vi "Set_init_data.vi"(8 "error in (no error)":errorcluster, 11 "HIS in":refnum<class "HIS.lvclass">) -> (0 "error out":errorcluster, 3 "HIS out":refnum<class "HIS.lvclass">)   [LabVIEW 2018, in "HIS.lvclass"]
uses:
  HIS.lvclass
  C:/Users/Sergey Denisov/Documents/REPS/TRANCON/Classes/DATA/DATA.lvclass
  DATA.lvclass/DATA.ctl
  Write width, pixels.vi
  Write height, pixels.vi
  DATA.lvclass
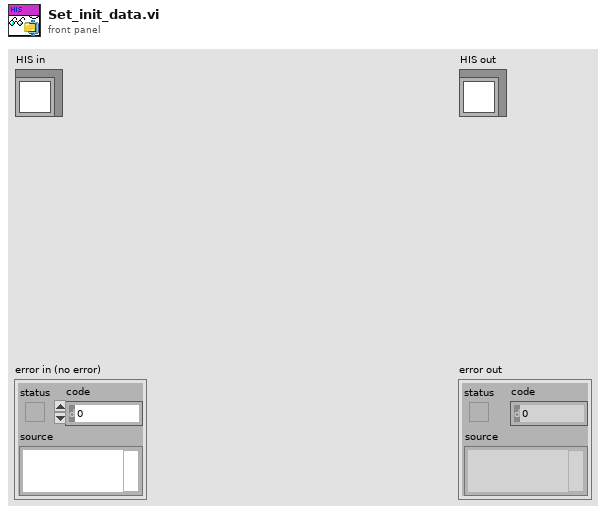
[diagram p1: front panel]
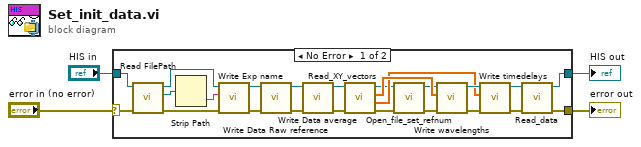
[diagram p0: block diagram]
diagram:
  n1 = case shown="No Error" "error in (no error)" {
    selector: "error in (no error)" -> [w28 w30]
    tunnel: [w5 w30] -> w3
    tunnel: "HIS in" -> [w27 w29]
    tunnel: [w6 w29] -> w1
    frame No Error {
      n2 = call "Read FilePath.vi"("error in (no error)"=w28, "DATA in"=w27) -> ("error out"=w25:errorcluster, "FilePath"=w24:path, "DATA out"=w22:refnum<class "HIS.lvclass">)  [unwired: 7 in]
      n3 = Strip Path(path=w24) -> (name=w23:string)  [unwired: 1 out]
      n4 = call "Write Exp name.vi"("error in (no error)"=w25, "Exp name"=w23, "DATA in"=w22) -> ("error out"=w20:errorcluster, "DATA out"=w19:refnum<class "HIS.lvclass">)  [unwired: 7 in]
      n5 = call "Write Data Raw reference.vi"("error in (no error)"=w20, "DATA in"=w19) -> ("error out"=w18:errorcluster, "DATA out"=w17:refnum<class "HIS.lvclass">)  [unwired: 8 in]
      n6 = call "Write Data average.vi"("error in (no error)"=w18, "DATA in"=w17) -> ("error out"=w16:errorcluster, "DATA out"=w15:refnum<class "HIS.lvclass">)  [unwired: 8 in]
      n7 = call-dynamic "Read_XY_vectors.vi"("error in (no error)"=w16, "HIS in"=w15) -> ("error out"=w12:errorcluster, "timedelays"=w13:dbl[], "wavelengths"=w14:dbl[], "HIS out"=w11:refnum<class "HIS.lvclass">)  [unwired: 6 in]
      n8 = call-dynamic "Open_file_set_refnum.vi"("error in (no error)"=w12, "DATA in"=w11) -> ("error out"=w10:errorcluster, "DATA out"=w9:refnum<class "HIS.lvclass">)  [unwired: 8 in]
      n9 = call "Write wavelengths.vi"("error in (no error)"=w10, "wavelengths"=w14, "DATA in"=w9) -> ("error out"=w26:errorcluster, "DATA out"=w21:refnum<class "HIS.lvclass">)  [unwired: 7 in]
      n10 = call "Write timedelays.vi"("error in (no error)"=w26, "timedelays"=w13, "DATA in"=w21) -> ("error out"=w8:errorcluster, "DATA out"=w7:refnum<class "HIS.lvclass">)  [unwired: 7 in]
      n11 = call-dynamic "Read_data.vi"("error in (no error)"=w8, "HIS IN"=w7) -> ("error out"=w5:errorcluster, "HIS OUT"=w6:refnum<class "HIS.lvclass">)  [unwired: 8 in]
    }
    frame Error {
    }
  }
  "error out" <- w3
  "HIS out" <- w1
